vi "N4_201_WriteAndCheck.vi"(4 "Driver Name":T9, 5 "Command Time (s)":T6=3.0, 6 "Error Code":T10, 7 "Command":T7, 8 "error in":T8, 11 "DriverConnect in":T1={"InterfaceType"=enum."VISA", "OpenedSession"="", "InterfaceSettings"={"Interface"=enum."RS232", "EOS 4 read"=enum."LF (\\n)", "EOS 4 write"=enum."LF (\\n)", "TMO, ms"=10000, "Sett"=variant(cluster{"Baud Rate":u32, "Data Bits":u16, "Parity":u16, "Stop Bits":u16, "Flow Control":u16, "Eho":bool} {"Baud Rate"=75, "Data Bits"=0, "Parity"=0, "Stop Bits"=0, "Flow Control"=0, "Eho"=FALSE})}}) -> (0 "error out":T8, 3 "DriverConnect out":T1={"InterfaceType"=enum."VISA", "OpenedSession"="", "InterfaceSettings"={"Interface"=enum."RS232", "EOS 4 read"=enum."LF (\\n)", "EOS 4 write"=enum."LF (\\n)", "TMO, ms"=10000, "Sett"=variant(cluster{"Baud Rate":u32, "Data Bits":u16, "Parity":u16, "Stop Bits":u16, "Flow Control":u16, "Eho":bool} {"Baud Rate"=75, "Data Bits"=0, "Parity"=0, "Stop Bits"=0, "Flow Control"=0, "Eho"=FALSE})}})   [LabVIEW 2018]
uses:
  MOKO_LabViewLibrary/MokoLowLevel/MokoLowLovelControl/MLLC_ErrorCode.ctl
  MOKO_LabViewLibrary/MokoLowLevel/MokoLowLovelControl/MLLC_DriverName.ctl
  MOKO_LabViewLibrary/MokoLowLevel/MokoLowLovelControl/MLLC_Error.ctl
  MOKO_LabViewLibrary/MokoLowLevel/MokoLowLovelControl/MLLC_Command.ctl
  MOKO_LabViewLibrary/MokoLowLevel/MokoLowLovelControl/MLLC_Delay.ctl
  MOKO_LabViewLibrary/MokoLowLevel/MokoLowLovelControl/MLLC_ConnectCluster.ctl
  MOKO_LabViewLibrary/MokoLowLevel/MokoLowLovelControl/MLLC_InterfaceType.ctl
  MOKO_LabViewLibrary/MokoLowLevel/MokoLowLovelControl/MLLC_OpenedSession.ctl
  MOKO_LabViewLibrary/MokoLowLevel/MokoLowLovelControl/MLLC_InterfaceSettings.ctl
  MOKO_LabViewLibrary/MokoLowLevel/MokoLowLovelControl/MLLC_InterfaceKind.ctl
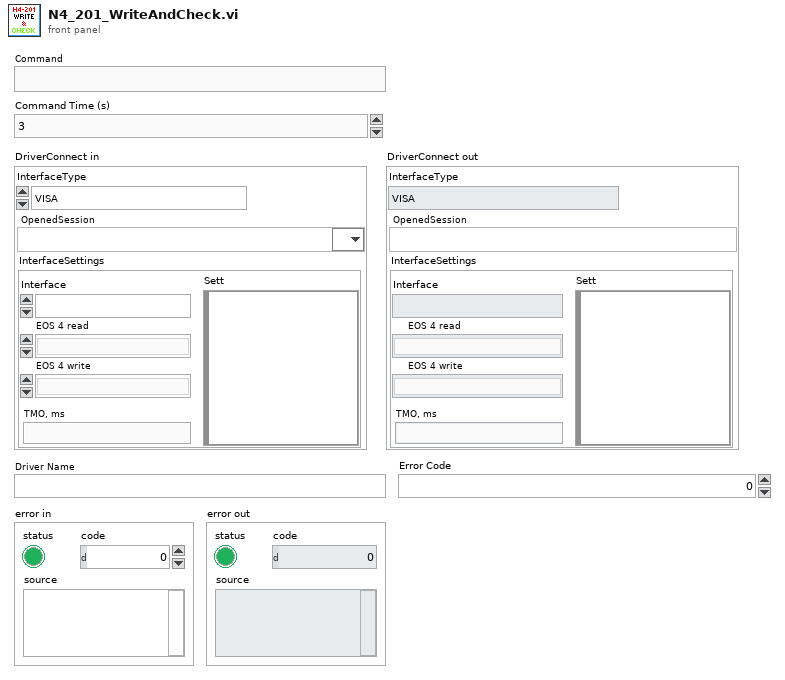
[diagram p1: front panel]
types:
  T1 = typedef "MLLC_ConnectCluster.ctl" = cluster{"InterfaceType":T2, "OpenedSession":T3, "InterfaceSettings":T4}
  T2 = typedef "MLLC_InterfaceType.ctl" = enum16{"VISA", "Prologix USB-GPIB"}
  T3 = typedef "MLLC_OpenedSession.ctl" = refnum<visa-resource-name>
  T4 = typedef "MLLC_InterfaceSettings.ctl" = cluster{"Interface":T5, "EOS 4 read":enum16{"Default (=EOS 4 write)", "CR (\\r)", "LF (\\n)", "None"}, "EOS 4 write":enum16{"CR+LF (\\r\\n)", "CR (\\r)", "LF (\\n)", "None"}, "TMO, ms":i32, "Sett":variant}
  T5 = typedef "MLLC_InterfaceKind.ctl" = enum16{"RS232", "GPIB", "USB", "Ethernet", "another"}
  T6 = typedef "MLLC_Delay.ctl" = dbl
  T7 = typedef "MLLC_Command.ctl" = string
  T8 = typedef "MLLC_Error.ctl" = errorcluster
  T9 = typedef "MLLC_DriverName.ctl" = string
  T10 = typedef "MLLC_ErrorCode.ctl" = u32
  T11 = enum16{"Нет симуляции", "В ручную", "Игнорировать"}
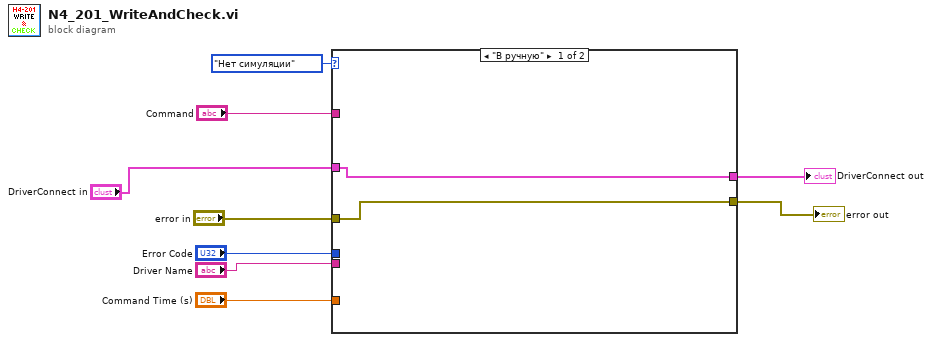
[diagram p0: block diagram]
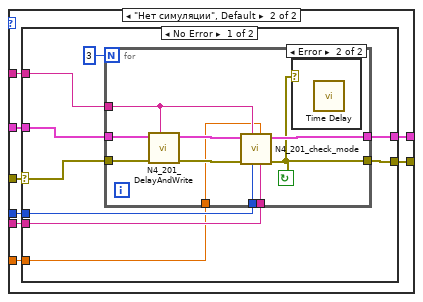
[diagram p2: hidden frame]
diagram:
  n1 = case shown="\"В ручную\"" T11."Нет симуляции" ("Simmulation") {
    tunnel: [w10 w19] -> w9
    tunnel: [w11 w18] -> w1
    tunnel: "Error Code" -> [_ w17]
    tunnel: "Driver Name" -> [_ w16]
    tunnel: "DriverConnect in" -> [w11 w15]
    tunnel: "error in" -> [w10 w14]
    tunnel: "Command" -> [_ w13]
    tunnel: "Command Time (s)" -> [_ w12]
    frame "В ручную" {
    }
    frame "Нет симуляции", Default {
      n2 = case shown="No Error" w14 {
        selector: w14 -> [w22 w40]
        tunnel: [w23 w40] -> w19
        tunnel: [w24 w39] -> w18
        tunnel: w17 -> [w26 _]
        tunnel: w16 -> [w25 _]
        tunnel: w15 -> [w27 w39]
        tunnel: w13 -> [w28 _]
        tunnel: w12 -> [w21 _]
        frame No Error {
          n3 = for {
            N: 3 -> [_]
            tunnel: w28 -> [w37]
            tunnel: w27 -> [w36]
            tunnel: w26 -> [w35]
            tunnel: w25 -> [w34]
            tunnel: [w33] -> w24
            tunnel: [w29] -> w23
            tunnel: w22 -> [w31]
            tunnel: w21 -> [w30]
            stop <- w29 continue-if-true
            n4 = call "N4_201_DelayAndWrite.vi"("Command"=w37, "error in"=w31, "DriverConnect in"=w36) -> ("error out"=w32:T8, "DriverConnect out"=w38:T1)  [unwired: 7 in]
            n5 = call "N4_201_check_mode.vi"("Driver Name"=w34, "Delay befor,s"=w30, "Error Code"=w35, "InputParam"=w37, "error in"=w32, "DriverConnect in"=w38) -> ("error out"=w29:T8, "DriverConnect out"=w33:T1)  [unwired: 4 in]
            n6 = case shown="Error" w29 {
              frame No Error {
              }
              frame Error {
                n7 = call "Time Delay"() -> ()  [unwired: 11 in, 1 out]
              }
            }
          }
        }
        frame Error {
        }
      }
    }
  }
  "error out" <- w9
  "DriverConnect out" <- w1
